vi "loadDataPerChannel.vi"(8 "error in (no error)":errorcluster, 10 "data":dbl[][][](array[numeric]), 11 "AnalogOutput in":refnum<class "AnalogOutput.lvclass">) -> (0 "error out":errorcluster, 3 "AnalogOutput out":refnum<class "AnalogOutput.lvclass">)   [LabVIEW 2009, in "Hardware.lvlib" / "Channels.lvlib" / "AnalogOutput.lvclass"]
uses:
  AnalogOutput.lvclass
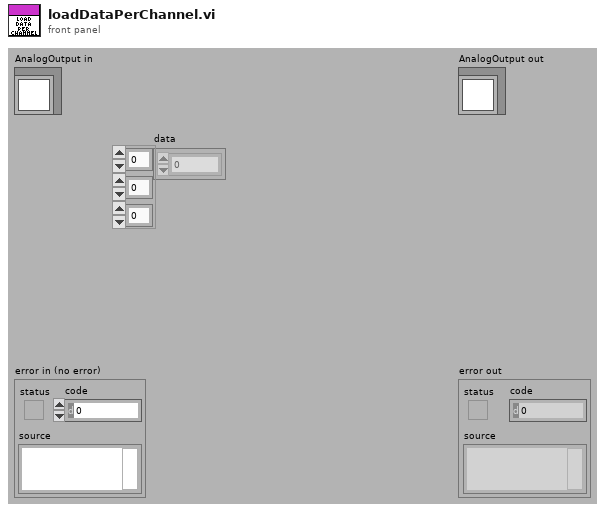
[diagram p1: front panel]
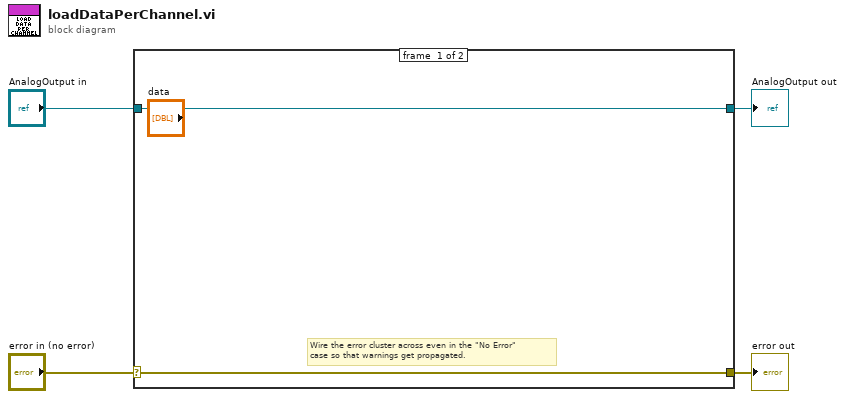
[diagram p0: block diagram]
diagram:
  n1 = case shown="No Error" "error in (no error)" {
    selector: "error in (no error)" -> [w5 w8]
    tunnel: [w5 w8] -> w3
    tunnel: [w6 w7] -> w1
    tunnel: "AnalogOutput in" -> [w6 w7]
    frame #0 {
      # "Wire the error cluster across even in the \"No Error\"\ncase so that warnings get propagated."
    }
    frame #1 {
    }
  }
  "error out" <- w3
  "AnalogOutput out" <- w1
